vi "Write Amplitude.vi"(8 "error in (no error)":errorcluster, 10 "Amplitude":dbl, 11 "SRS_SG380 in":refnum<class "SRS_SG380.lvclass">) -> (0 "error out":errorcluster, 3 "SRS_SG380 out":refnum<class "SRS_SG380.lvclass">)   [LabVIEW 2013, in "SRS_SG380.lvclass"]
uses:
  SRS_SG380.lvclass
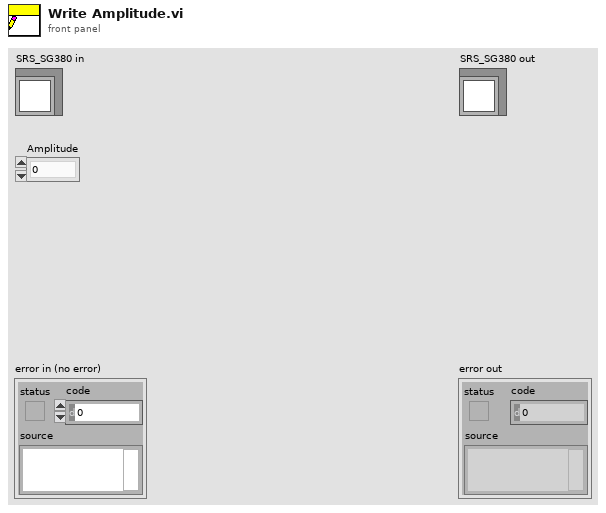
[diagram p1: front panel]
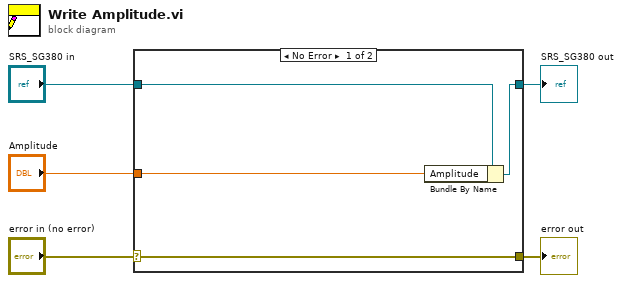
[diagram p0: block diagram]
diagram:
  n1 = case shown="No Error" "error in (no error)" {
    selector: "error in (no error)" -> [w9 w10]
    tunnel: [w9 w10] -> w4
    tunnel: [w7 w11] -> w2
    tunnel: "SRS_SG380 in" -> [w8 w11]
    tunnel: "Amplitude" -> [w6 _]
    frame No Error {
      n2 = Bundle By Name(cluster=w8, "Amplitude"=w6) -> (w7:refnum<class "SRS_SG380.lvclass">)
    }
    frame Error {
    }
  }
  "error out" <- w4
  "SRS_SG380 out" <- w2
